vi "Execute Command.vi"(8 "error in (no error)":errorcluster, 10 "Slide Panel On Screen in":refnum<class "Slide Panel On Screen.lvclass">, 11 "User Interface References":T1={"This VI"=refnum, "User Interace Plugin"=refnum, "UI Picture Container References"={"Header Image"=refnum, "Footer Image"=refnum}, "Sliding Menu XControl"=refnum, "Menu Container"=refnum, "UI Configuration Information"={"Space Between Buttons"=3, "Number of Buttons to Show"=6, "Header Image"=path "Images/Blue Background.bmp", "Footer Image"=path "Images/Blue Background.bmp"}, "Header Text"=refnum}) -> (0 "error out":errorcluster, 1 "Stop?":bool, 2 "Slide Panel On Screen out":refnum<class "Slide Panel On Screen.lvclass">, 3 "User Interface References Out":T1={"This VI"=refnum, "User Interace Plugin"=refnum, "UI Picture Container References"={"Header Image"=refnum, "Footer Image"=refnum}, "Sliding Menu XControl"=refnum, "Menu Container"=refnum, "UI Configuration Information"={"Space Between Buttons"=3, "Number of Buttons to Show"=6, "Header Image"=path "Images/Blue Background.bmp", "Footer Image"=path "Images/Blue Background.bmp"}, "Header Text"=refnum})   [LabVIEW 2011, in "Slide Panel On Screen.lvclass"]
uses:
  Slide Panel On Screen.lvclass
  Main Type Definitions/User Interface Type Definitions.ctl
  Main Type Definitions/UI Picture Containers.ctl
  Sliding Menu/Sliding Menu Library/Sliding Menu xControl/Sliding Menu XControl.xctl
  UI Control Definitions/UI Configuration Information.ctl
  Plugin Handler/Plugin Command Manager/Notify Plugin Slide Complete/Notify Plugin Slide Completed.lvclass
  <vilib>/Utility/miscctls.llb/LVPositionTypeDef.ctl
  UI Slide Panel/Slide Panel Off Screen.lvclass
  Plugin Handler/Plugin Command Manager/Plugin Handler Command.lvclass
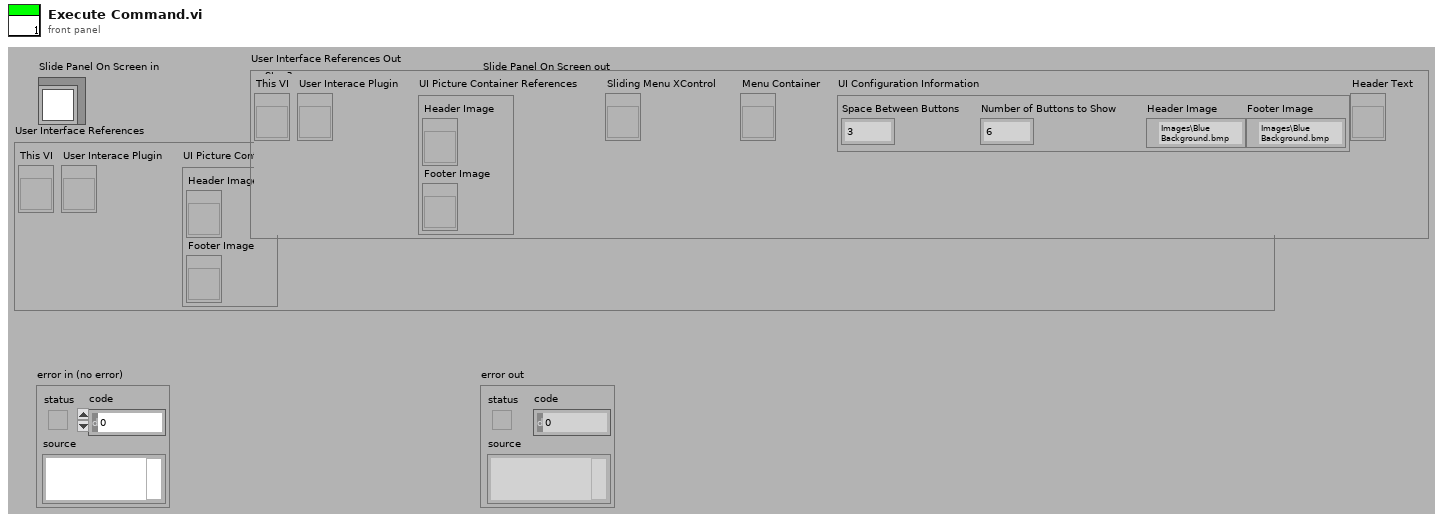
[diagram p1: front panel]
types:
  T1 = typedef "User Interface Type Definitions.ctl" = cluster{"This VI":refnum<vi>, "User Interace Plugin":refnum<vi>, "UI Picture Container References":T2, "Sliding Menu XControl":refnum<vi>, "Menu Container":refnum<vi>, "UI Configuration Information":T3, "Header Text":refnum<vi>}
  T2 = typedef "UI Picture Containers.ctl" = cluster{"Header Image":refnum<vi>, "Footer Image":refnum<vi>}
  T3 = typedef "UI Configuration Information.ctl" = cluster{"Space Between Buttons":i32, "Number of Buttons to Show":i32, "Header Image":path, "Footer Image":path}
  T4 = typedef "LVPositionTypeDef.ctl" = cluster{"Left":i32, "Top":i32}
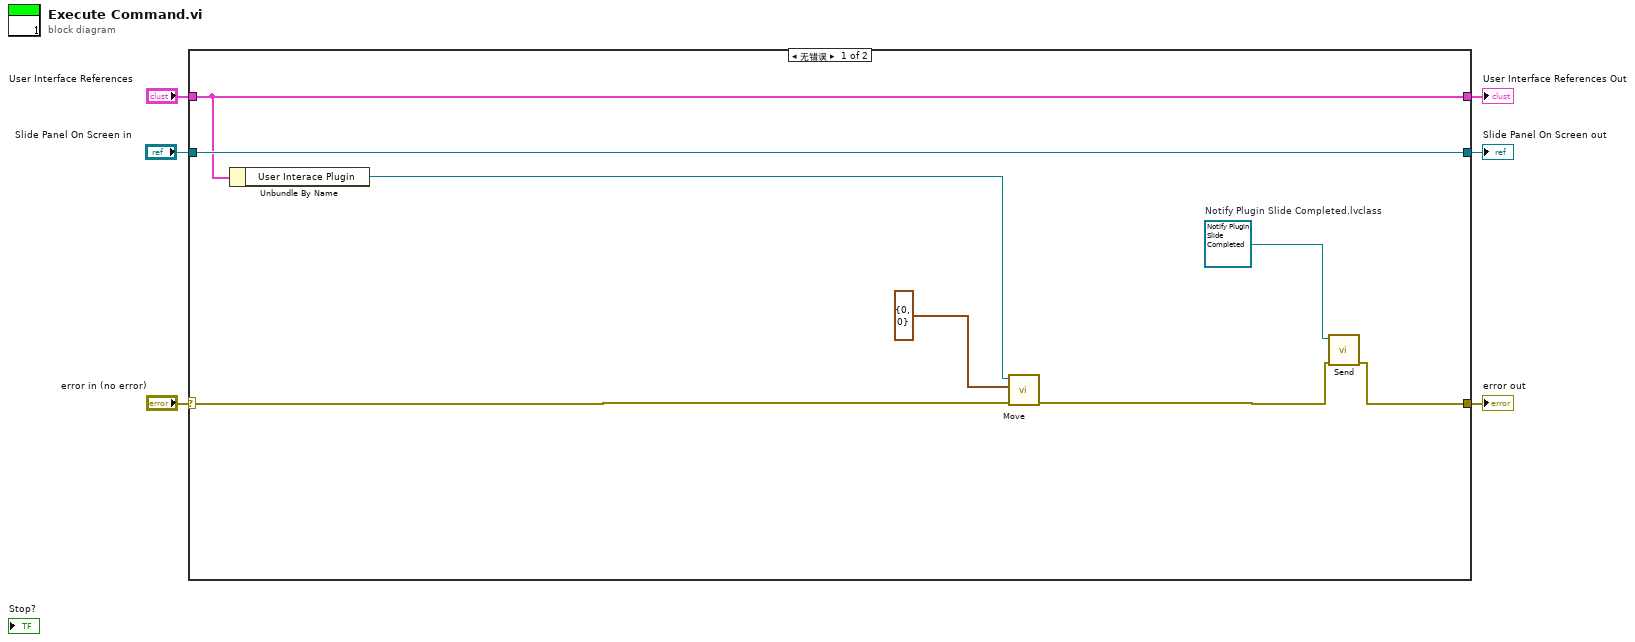
[diagram p0: block diagram]
diagram:
  n1 = case shown="无错误" "error in (no error)" {
    selector: "error in (no error)" -> [w10 w15]
    tunnel: [w13 w17] -> w1
    tunnel: "User Interface References" -> [w13 w17]
    tunnel: [w14 w16] -> w2
    tunnel: "Slide Panel On Screen in" -> [w14 w16]
    tunnel: [w7 w15] -> w3
    frame No Error {
      w9 = refnum<class "Notify Plugin Slide Completed.lvclass"> refnum  # Notify Plugin Slide Completed.lvclass
      n2 = Unbundle By Name(w13) -> ("User Interace Plugin"=w12:refnum<vi>)
      n3 = call "Move.vi"("error in (no error)"=w10, "Desired Position"=T4 {"Left"=0, "Top"=0}, "Obj Ref"=w12) -> ("error out"=w8:errorcluster)  [unwired: 6 in, 2 out]
      n4 = call "Send.vi"("error in (no error)"=w8, "Plugin Generic Command in"=w9) -> ("error out"=w7:errorcluster)  [unwired: 8 in, 1 out]
    }
    frame Error {
    }
  }
  "error out" <- w3
  "Slide Panel On Screen out" <- w2
  "User Interface References Out" <- w1
